vi "Find_Unique_Filename.vi"(0 "Path In":path, 1 "Max Length (31)":i32=31) -> (3 "Unique Path Out":path)   [LabVIEW 2015]
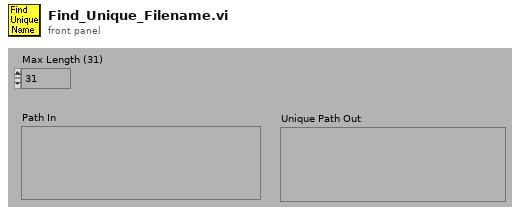
[diagram p1: front panel]
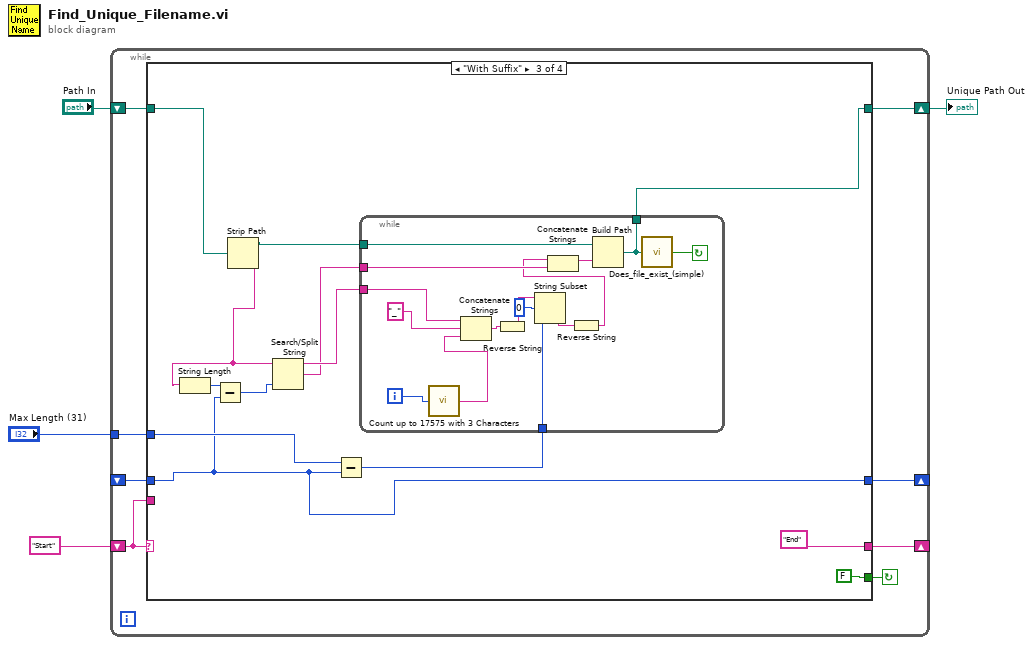
[diagram p0: block diagram]
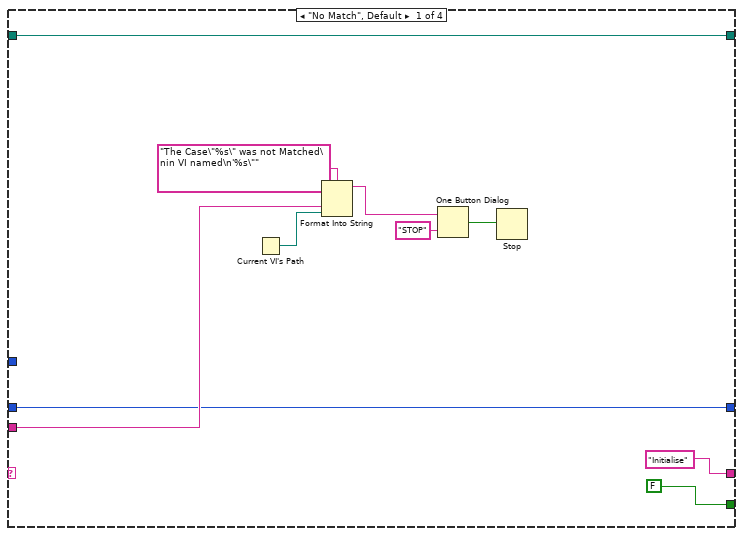
[diagram p2: hidden frame]
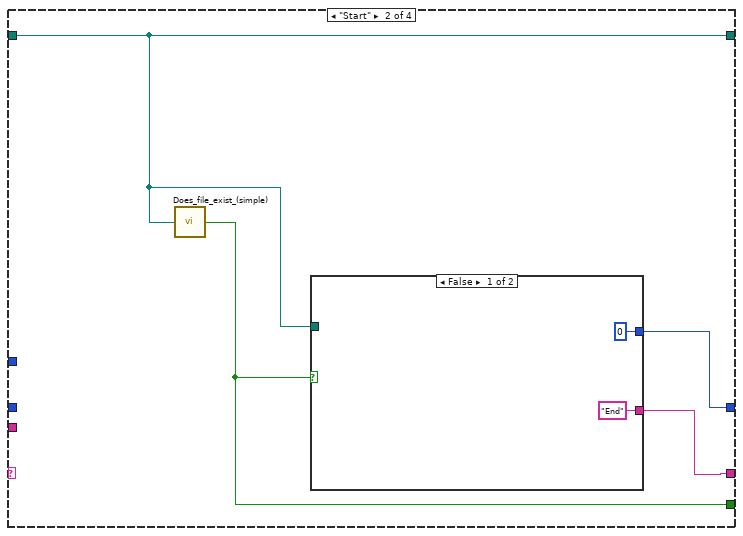
[diagram p3: hidden frame]
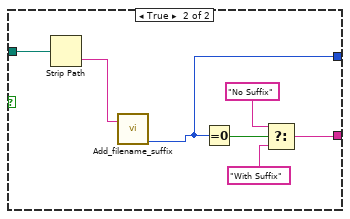
[diagram p4: hidden frame]
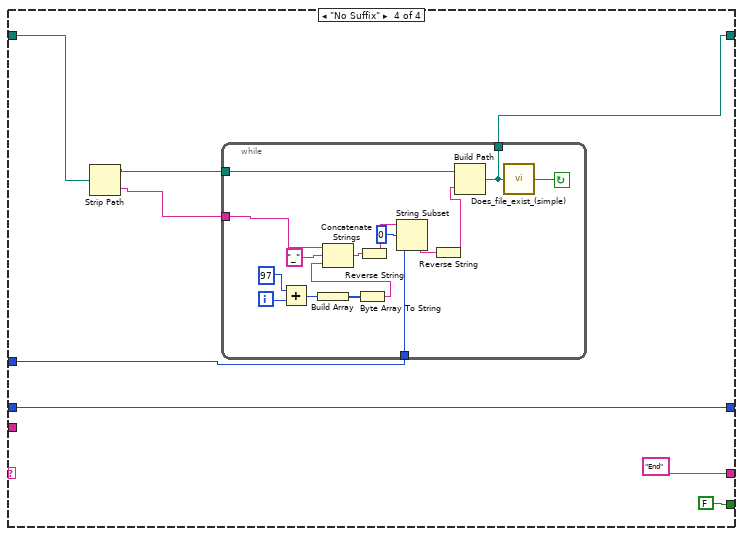
[diagram p5: hidden frame]
diagram:
  n1 = while {
    shift-left: "Start" -> [w10]
    shift-right: [w11] -> _
    shift-right: [w8] -> w2
    shift-left: "Path In" -> [w9]
    tunnel: "Max Length (31)" -> [w7]
    shift-right: [w6] -> _
    shift-left: _ -> [w5]
    stop <- w12 continue-if-true
    n2 = case shown="\"With Suffix\"" w10 {
      tunnel: [FALSE w25 FALSE FALSE] -> w12
      tunnel: ["Initialise" w26 "End" "End"] -> w11
      tunnel: w10 -> [w17 _ _ _]
      tunnel: w9 -> [w14 w24 w41 w68]
      tunnel: [w14 w24 w40 w67] -> w8
      tunnel: w7 -> [_ _ w43 w65]
      tunnel: [w13 w23 w36 w64] -> w6
      tunnel: w5 -> [w13 _ w36 w64]
      frame "No Match", Default {
        n3 = Current VI's Path() -> (path=w16:path)
        n4 = Format Into String(format string="The Case\"%s\" was not Matched\nin VI named\n'%s\"" ("Format String"), w17, w16) -> (resulting string=w20:string)  [unwired: 2 in, 1 out]
        n5 = One Button Dialog(message=w20, button name ("OK")="STOP") -> (true=w18:bool)
        n6 = Stop(stop? (T)=w18) -> ()
      }
      frame "Start" {
        n7 = call "Does_file_exist_(simple).vi"("Pathname"=w24) -> ("exists?"=w25:bool)
        n8 = case shown="False" w25 {
          tunnel: ["End" w34] -> w26
          tunnel: w24 -> [_ w31]
          tunnel: [0 ("Extension length") w29] -> w23
          frame False {
          }
          frame True {
            n9 = Strip Path(path=w31) -> (name=w30:string)  [unwired: 1 out]
            n10 = call "Add_filename_suffix.vi"("Filename"=w30) -> ("Extension length"=w29:i32)  [unwired: 1 in, 3 out]
            n11 = Equal To 0?(x=w29) -> (x = 0?=w35:bool)
            n12 = Select(t="No Suffix", s=w35, f="With Suffix") -> (s? t:f=w34:string)
          }
        }
      }
      frame "With Suffix" {
        n13 = Strip Path(path=w41) -> (stripped path=w46:path, name=w45:string)
        n14 = String Length(string=w45) -> (length=w44:i32)
        n15 = Subtract(x=w44, y=w36) -> (x-y=w39:i32)
        n16 = Search/Split String(string=w45, offset (0)=w39) -> (substring before match=w38:string, match + rest of string=w37:string)  [unwired: 2 out]
        n17 = Subtract(x=w43, y=w36) -> (x-y=w42:i32)
        n18 = while {
          tunnel: w38 -> [w63]
          tunnel: w42 -> [w62]
          tunnel: w46 -> [w61]
          tunnel: w37 -> [w60]
          tunnel: [w52] -> w40
          i -> [w50]
          stop <- w53 continue-if-true
          n19 = call "Count up to 17575 with 3 Characters.vi"("Numeric Control"=w50) -> ("string"=w49:string)
          n20 = Concatenate Strings(w63, "_" ("string"), w49) -> (w58:string)
          n21 = Reverse String(1:w58) -> (0:w59:string)
          n22 = String Subset(string=w59, offset (0)=0, length (rest)=w62) -> (substring=w57:string)
          n23 = Reverse String(1:w57) -> (0:w55:string)
          n24 = Concatenate Strings(w55, w60) -> (w54:string)
          n25 = Build Path(base path=w61, name or relative path=w54) -> (appended path=w52:path)
          n26 = call "Does_file_exist_(simple).vi"("Pathname"=w52) -> ("exists?"=w53:bool)
        }
      }
      frame "No Suffix" {
        n27 = Strip Path(path=w68) -> (stripped path=w69:path, name=w66:string)
        n28 = while {
          tunnel: w66 -> [w87]
          tunnel: w65 -> [w86]
          tunnel: w69 -> [w85]
          tunnel: [w75] -> w67
          i -> [w77]
          stop <- w76 continue-if-true
          n29 = Add(x=97, y=w77) -> (x+y=w83:i32)
          n30 = Build Array(w83) -> (w84:i32[])
          n31 = Byte Array To String(unsigned byte array=w84) -> (string=w73:string)
          n32 = Concatenate Strings(w87, "_" ("string"), w73) -> (w80:string)
          n33 = Reverse String(1:w80) -> (0:w81:string)
          n34 = String Subset(string=w81, offset (0)=0, length (rest)=w86) -> (substring=w79:string)
          n35 = Reverse String(1:w79) -> (0:w74:string)
          n36 = Build Path(base path=w85, name or relative path=w74) -> (appended path=w75:path)
          n37 = call "Does_file_exist_(simple).vi"("Pathname"=w75) -> ("exists?"=w76:bool)
        }
      }
    }
  }
  "Unique Path Out" <- w2
